vi "CreateHDF5.vi"() -> (0 "error out":errorcluster, 3 "File Handle":T1=16777216 format="%.0x")   [LabVIEW 2014]
uses:
  <vilib>/addons/h5labview2/base/hid_t.ctl
panel:
  in  "Click OK when all data are entered.":bool
  in  "QDC Info, Ch0 - 7, left to right":T2={"Chanel Description"=["H0", "H1", "H2", "H3", "H4", "H5"], "Only Hodo?"=[TRUE, TRUE, TRUE, TRUE, TRUE, TRUE]}
  in  "Scaler Info":T2={"Chanel Description"=["H0", "H1", "H2", "H3", "H4", "H5", "TrigA", "TrigB", "TrigC", "TrigD", "Ch0", "Ch1", "Ch2", "Ch3", "Ch4", "Ch5", "Ch6", "Ch7"], "Only Hodo?"=[TRUE, TRUE, TRUE, TRUE, TRUE, TRUE, TRUE, TRUE, FALSE, FALSE, FALSE, FALSE, FALSE, FALSE, FALSE, FALSE, FALSE, FALSE]}
  in  "Digitizer Info, Ch0 - 4, left to right":T2={"Chanel Description"=["Ch0", "Ch1", "Ch2", "Ch3", "Ch4", "Ch5", "Ch6", "Ch7"], "Only Hodo?"=[FALSE, FALSE, FALSE, FALSE, FALSE, FALSE, FALSE, FALSE]}
  in  "TDC Info":T2={"Chanel Description"=["H0", "H1", "H2", "H3", "H4", "H5", "TrigA", "TrigB", "TrigC", "TrigD"], "Only Hodo?"=[TRUE, TRUE, TRUE, TRUE, TRUE, TRUE, TRUE, TRUE, FALSE, FALSE]}
  in  "Trigger Bit Descriptions":string[](array[string])=["TrigA", "TrigB", "TrigC", "TrigD"]
  in  "Thermocouple Location":string[](array[string])=["In Dark Box", "In Room"]
  in  "HDF5 File Path":path=path "C:/Users/lbignell/Desktop/dummy3.h5"
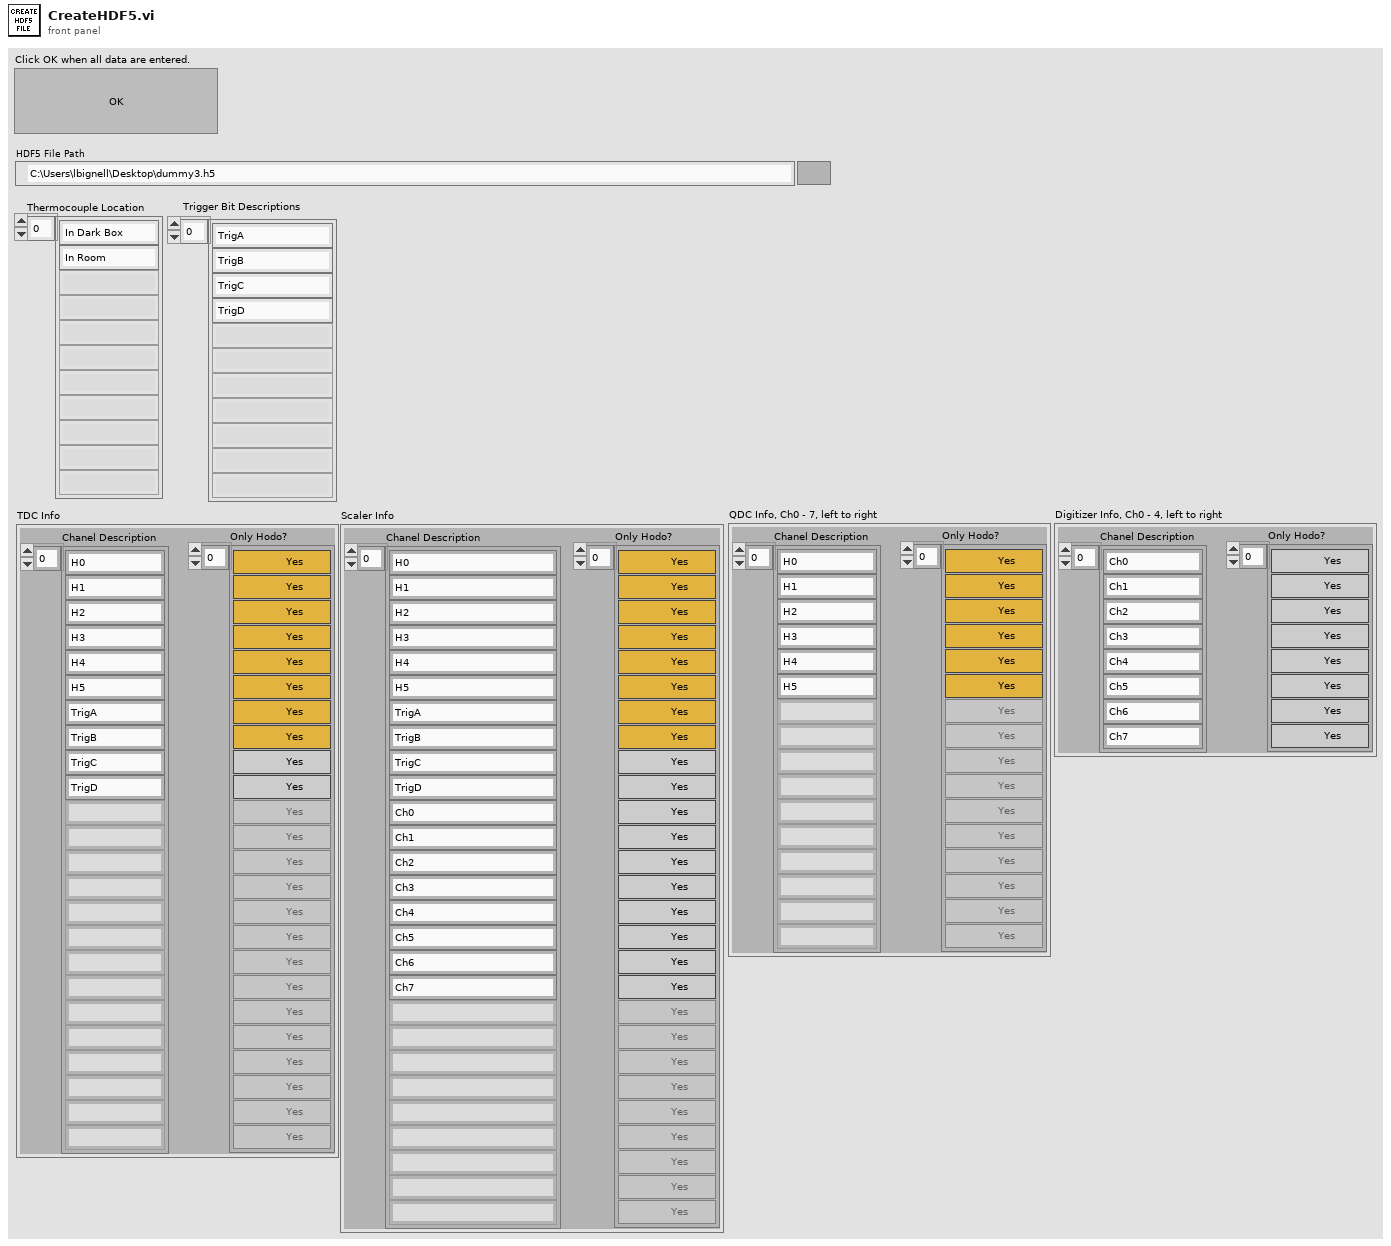
[diagram p1: front panel]
types:
  T1 = typedef "hid_t.ctl" = i32
  T2 = cluster{"Chanel Description":string[], "Only Hodo?":bool[]}
  T3 = cluster{"Module Description":string[], "Module Model":string[], "Module Address":u32[]}
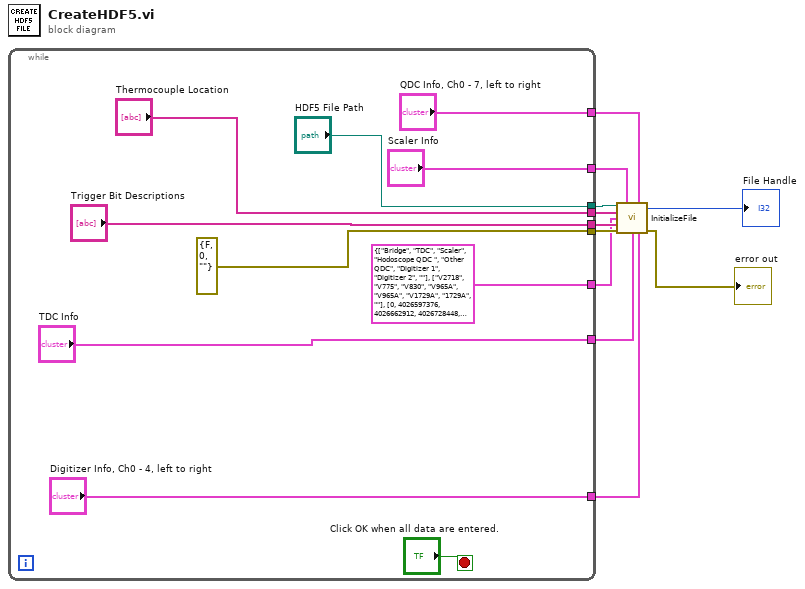
[diagram p0: block diagram]
diagram:
  n1 = while {
    tunnel: ["HDF5 File Path"] -> w11
    tunnel: [errorcluster {"status"=FALSE, "code"=0, "source"=""} ("error in")] -> w10
    tunnel: ["Thermocouple Location"] -> w9
    tunnel: ["Trigger Bit Descriptions"] -> w8
    tunnel: ["QDC Info, Ch0 - 7, left to right"] -> w7
    tunnel: ["Scaler Info"] -> w6
    tunnel: ["TDC Info"] -> w5
    tunnel: ["Digitizer Info, Ch0 - 4, left to right"] -> w4
    tunnel: [T3 {"Module Description"=["Bridge", "TDC", "Scaler", "Hodoscope QDC ", "Other QDC", "Digitizer 1", "Digitizer 2", ""], "Module Model"=["V2718", "V775", "V830", "V965A", "V965A", "V1729A", "1729A", ""], "Module Address"=[0, 4026597376, 4026662912, 4026728448, 4026793984, 4026859520, 4026925056]} ("VME Configuration")] -> w1
    stop <- "Click OK when all data are entered." stop-if-true
  }
  n2 = call "InitializeFile.vi"("File Path"=w11, "Scaler Info"=w6, "QDC Info"=w7, "Thermocouple Location"=w9, "VME Configuration"=w1, "Trigger Bit Descriptions"=w8, "error in"=w10, "TDC Info"=w5, "Digitizer Info"=w4) -> ("File Handle"=→"File Handle":T1, "error out"=→"error out":errorcluster)  [unwired: 5 in]
